vi "MSScript_Calc_UpdSourceArray.vi"(2 "ArrayVariable in":ext[](array[numeric]), 3 "VarString in":string) -> (0 "ArrayVariable out":ext[](array[numeric]), 1 "Cmd Error?":bool)   [LabVIEW 2018, in "MSScript.lvclass"]
uses:
  MSScript.lvclass
  MSScript_Transform_EXTArray.vi
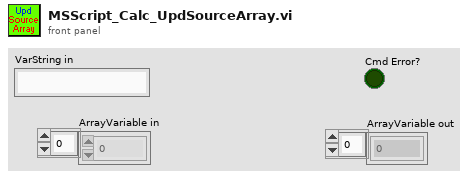
[diagram p1: front panel]
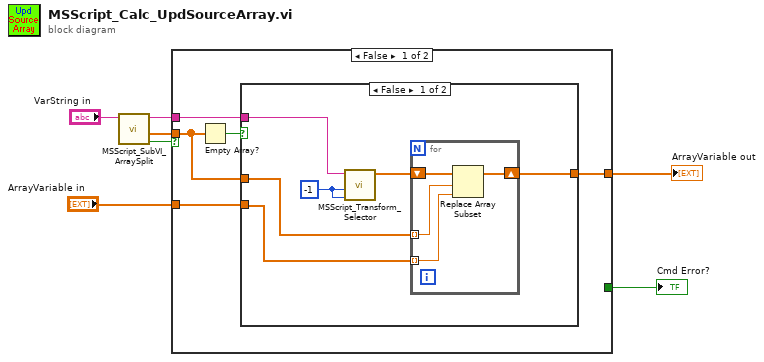
[diagram p0: block diagram]
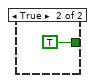
[diagram p3: hidden frame]
diagram:
  n1 = call "MSScript_SubVI_ArraySplit.vi"("VarString in"="VarString in") -> ("Value Error?"=w1:bool, "ArrayVariable out"=w3:ext[], "@name"=w2:string)  [unwired: 7 in, 1 out]
  n2 = case shown="False" w1 {
    tunnel: w3 -> [w9 _]
    tunnel: w2 -> [w11 _]
    tunnel: "ArrayVariable in" -> [w10 _]
    tunnel: [w8 _] -> w7
    tunnel: [_ TRUE] -> w5
    frame False {
      n3 = Empty Array?(array=w9) -> (empty?=w12:bool)
      n4 = case shown="False" w12 {
        tunnel: w11 -> [w14 _]
        tunnel: w10 -> [w15 w23]
        tunnel: w9 -> [w16 _]
        tunnel: [w13 w23] -> w8
        frame False {
          w18 = -1 ("MaxSize")
          n5 = call-poly "MSScript_Transform_Selector.vi"("MinSize"=w18, "MaxSize"=w18, "check_str"=w14) -> ("Value Output"=w17:ext[])  [unwired: 6 in, 2 out]
          n6 = for {
            tunnel: w16 -> [w21] mode=indexing
            tunnel: w15 -> [w20] mode=indexing
            shift-right: [w19] -> w13
            shift-left: w17 -> [w22]
            n7 = Replace Array Subset(array=w22, new element=w20, index=w21) -> (w19:ext[])
          }
        }
        frame True {
        }
      }
    }
    frame True {
    }
  }
  "ArrayVariable out" <- w7
  "Cmd Error?" <- w5
